vi "Gitlab OAuth Test.vi"() -> ()   [LabVIEW 2013]
uses:
  source/Oauth2/Oauth2.lvclass/Oauth2.ctl
  source/Oauth2/Read RefreshToken.vi
  source/Oauth2/Read ExpiresIn.vi
  source/Oauth2/Read Redirect URI.vi
  source/Oauth2/Read scopes.vi
  <vilib>/dlg_ctls.llb/Space Constant.vi
  source/OAuthToken/Retrieve Element.vi
  source/Oauth2.GitLab/Read Created At.vi
  source/Oauth2.GitLab/Read Created Timestamp.vi
  source/Oauth2/Oauth2.lvclass
  source/Oauth2.GitLab/Oauth2.GitLab.lvclass
  <vilib>/LabVIEW Open Source Project/OpenURI/uri/URI.lvclass
  <vilib>/httpClient/LabVIEWHTTPClient.lvlib
panel:
  out "REST API Error":errorcluster
  in  "Query API Version":bool
  in  "Refresh":bool
  in  "Authorize":bool
  out "Gitlab Version":string
  out "HTTP Response Headers":string
  out "Redirect URI":string
  out "granted scopes":string[](array[string])
  out "Created At":u32
  out "Expires In":u32
  out "Refresh Token":string
  in  "GitLab Client Secret":string
  in  "GitLab Client ID":string
  out "GitLab Access Token":string
  out "Oauth Error":errorcluster
  in  "GitLab Authorization Server URI":string="https://gitlab.com"
  # "Gitlab Application API Access Example"
  # "G Open Source Project for LabVIEW\nhttps://github.com/LabVIEW-Open-Source/Oauth2"
  # "1- Get a Client ID and Client Secret from the application's admin. \n\n          * To access your own server, log into your site, create an application and set the access scope.\n             you want. \n          * This Oauth2.0 API uses the following redirect URL: http://localhost:58888/Oauth2/Redirect\n          * Record the client ID and client secret and fill in the fields below."
  # "2- Set the Gitlab Authorization server address, without the relative \"oauth/authorize\" path.\n         * If using Gitlab's cloud, the URI is \"https://gitlab.com\"\n         * With your own domain, it could be \"https://gitlab.example.com\" or something similar."
  # "0: Never expired"
  # "3- Get an Access Token. You will be redirected your Gitlab's Authorization Server URI\n              * Use the \"Get Access Token\" button on the top right of this page.\n\n4- Once you have authenticated yourself, you will receive an access token.\n              * Use the \"Refresh Token\" button to request a fresh token\n                       OR\n              * Use the Access Token to query the Gitlab API (example is to retrieve the Gitlab Version)"
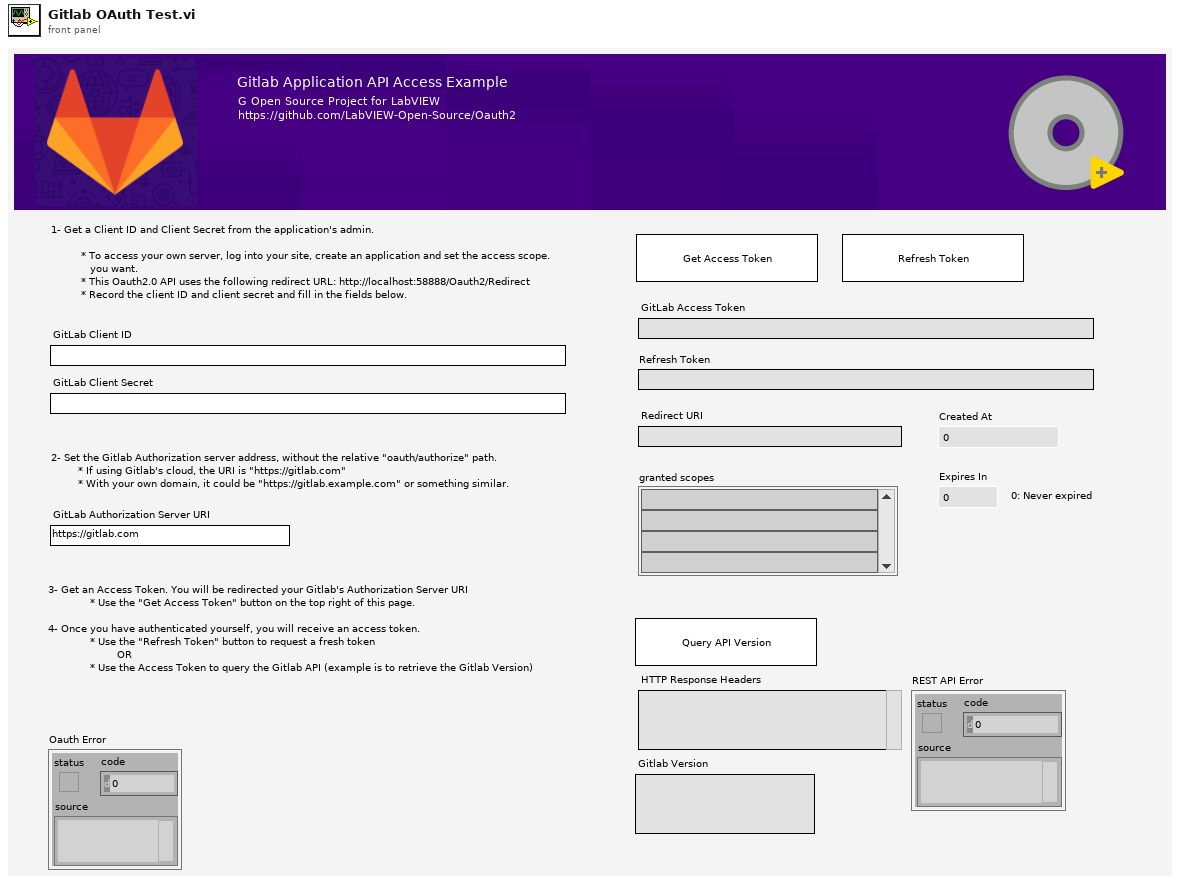
[diagram p1: front panel]
types:
  T1 = enum8{"Enabled", "Disabled", "Disabled and Grayed Out"}
  T2 = cluster{"Oauth2.GitLab":refnum<class "Oauth2.GitLab.lvclass">, "GitLab Authorization Server URI":string}
  T3 = typedef "LabVIEWHTTPClient.lvlib/ClientHandle.ctl" = refnum<k1>
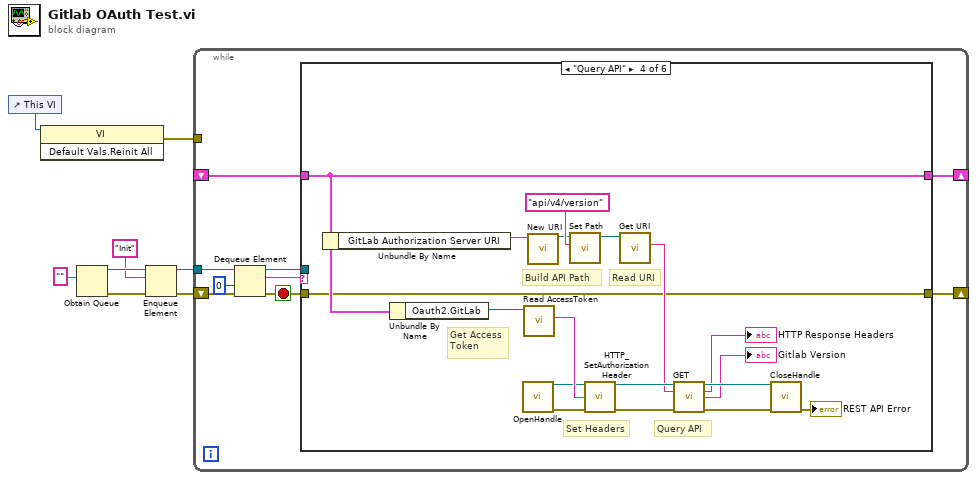
[diagram p0: block diagram]
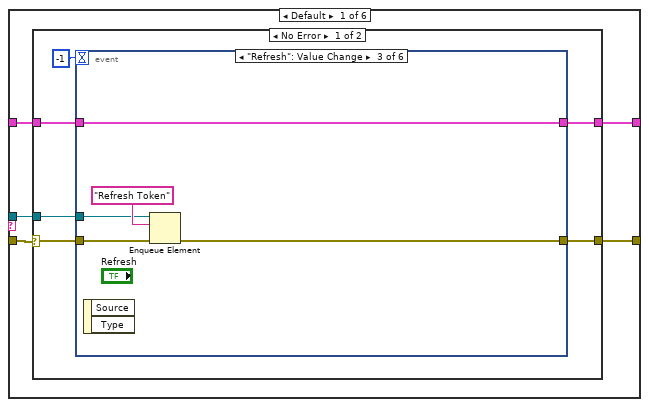
[diagram p2: hidden frame]
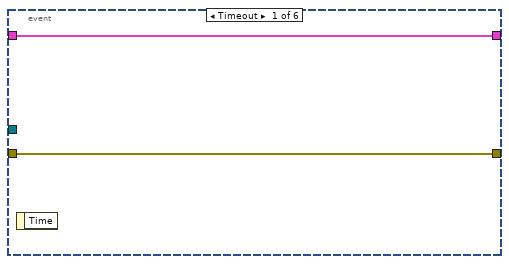
[diagram p3: hidden frame]
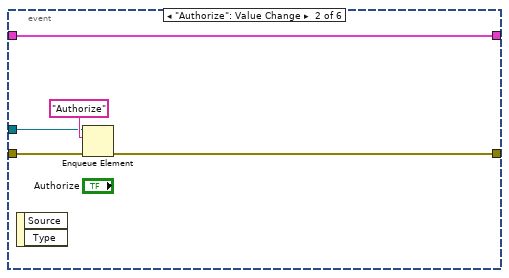
[diagram p4: hidden frame]
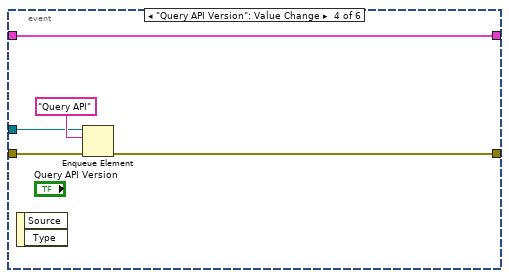
[diagram p5: hidden frame]
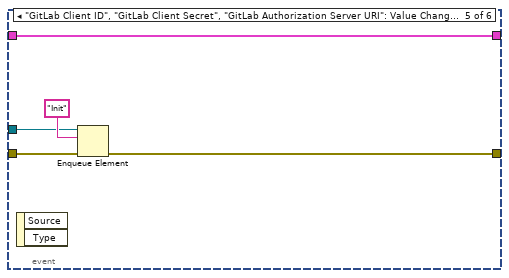
[diagram p6: hidden frame]
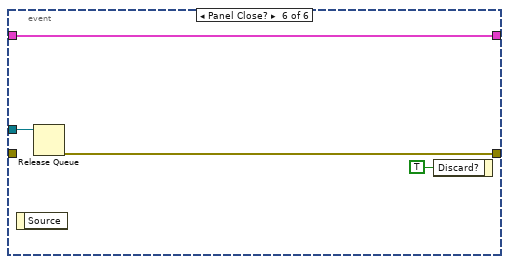
[diagram p7: hidden frame]
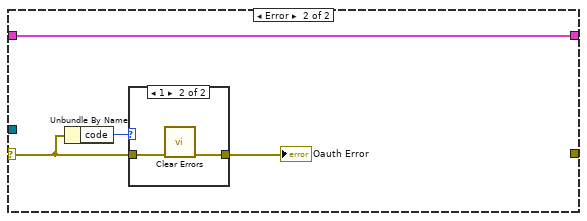
[diagram p8: hidden frame]
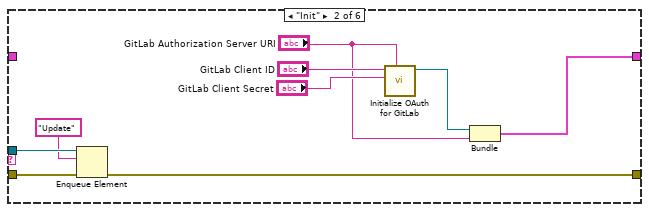
[diagram p10: hidden frame]
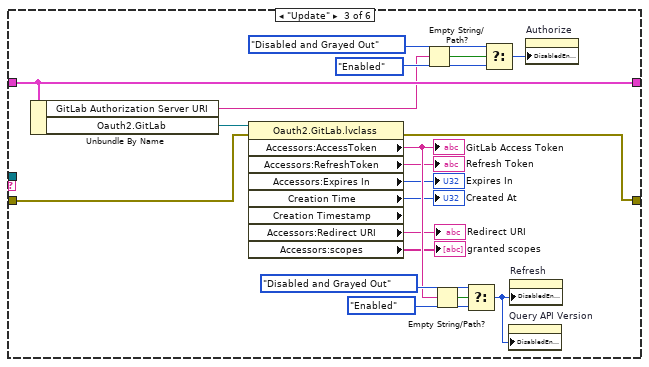
[diagram p11: hidden frame]
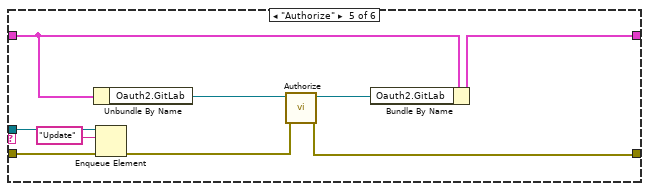
[diagram p12: hidden frame]
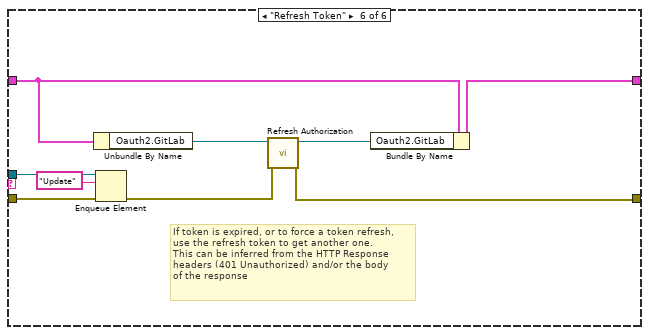
[diagram p13: hidden frame]
diagram:
  n1 = control-ref of="This VI"() -> (w2:refnum<vi>)
  n2 = invoke class="VI" method="Default Vals.Reinit All"(reference=w2) -> (error out=w1:errorcluster)  [unwired: 2 in, 2 out]
  n3 = Obtain Queue(element data type="") -> (queue out=w5:refnum<queue>, error out=w7:errorcluster)  [unwired: 4 in, 1 out]
  n4 = Enqueue Element(queue=w5, element="Init", error in (no error)=w7) -> (queue out=w4:refnum<queue>, error out=w6:errorcluster)  [unwired: 1 in, 1 out]
  n5 = while {
    tunnel: w4 -> [w17]
    shift-right: [w12] -> _
    shift-left: _ -> [w11]
    shift-right: [w9] -> _
    shift-left: w6 -> [w13]
    tunnel: w1 -> [_]
    stop <- w10 stop-if-true
    n6 = Dequeue Element(queue=w17, timeout in ms (-1)=0, error in (no error)=w13) -> (queue out=w14:refnum<queue>, element=w15:string, error out=w10:errorcluster)  [unwired: 1 out]
    n7 = case shown="\"Query API\"" w15 {
      tunnel: w14 -> [w22 w69 _ _ w110 w122]
      tunnel: [w21 w70 w89 w104 w112 w124] -> w12
      tunnel: w11 -> [w20 _ w89 w104 w113 w125]
      tunnel: w10 -> [w19 w66 w79 w92 w109 w121]
      tunnel: [w18 w67 w78 w92 w115 w117] -> w9
      frame Default {
        n8 = case shown="No Error" w19 {
          selector: w19 -> [w23 w57]
          tunnel: w22 -> [w27 _]
          tunnel: [w26 w58] -> w21
          tunnel: w20 -> [w25 w58]
          tunnel: [w24 _] -> w18
          frame No Error {
            n9 = event shown="[2] \"Refresh\": Value Change" {
              selector: _ -> [_ _ _ _ _ _]
              dyn-events: _ -> [_ _ _ _ _ _]
              timeout: -1 -> [_ _ _ _ _ _]
              tunnel: w27 -> [_ w34 w39 w44 w49 w54]
              tunnel: [w30 w32 w37 w42 w47 w52] -> w26
              tunnel: w25 -> [w30 w32 w37 w42 w47 w52]
              tunnel: [w29 w31 w36 w41 w46 w51] -> w24
              tunnel: w23 -> [w29 w33 w38 w43 w48 _]
              event Timeout {
                n10 = event-data() -> ()  [unwired: 1 in, 1 out]
              }
              event "Authorize": Value Change {
                n11 = event-data() -> ()  [unwired: 1 in, 2 out]
                n12 = Enqueue Element(queue=w34, element="Authorize", error in (no error)=w33) -> (error out=w31:errorcluster)  [unwired: 1 in, 2 out]
              }
              event "Refresh": Value Change {
                n13 = event-data() -> ()  [unwired: 1 in, 2 out]
                n14 = Enqueue Element(queue=w39, element="Refresh Token", error in (no error)=w38) -> (error out=w36:errorcluster)  [unwired: 1 in, 2 out]
              }
              event "Query API Version": Value Change {
                n15 = event-data() -> ()  [unwired: 1 in, 2 out]
                n16 = Enqueue Element(queue=w44, element="Query API", error in (no error)=w43) -> (error out=w41:errorcluster)  [unwired: 1 in, 2 out]
              }
              event "GitLab Client ID", "GitLab Client Secret", "GitLab Authorization Server URI": Value Change {
                n17 = event-data() -> ()  [unwired: 1 in, 2 out]
                n18 = Enqueue Element(queue=w49, element="Init", error in (no error)=w48) -> (error out=w46:errorcluster)  [unwired: 1 in, 2 out]
              }
              event Panel Close? {
                n19 = event-data() -> ()  [unwired: 1 in, 1 out]
                n20 = Release Queue(queue=w54) -> (error out=w51:errorcluster)  [unwired: 2 in, 2 out]
                n21 = event-data("Discard?"=TRUE) -> ()  [unwired: 1 in, 1 out]
              }
            }
          }
          frame Error {
            n22 = Unbundle By Name(w57) -> ("code"=w55:i32)
            n23 = case shown="1" w55 {
              tunnel: w57 -> [w59 w61]
              tunnel: [w59 w60] -> w56
              frame Default {
              }
              frame 1 {
                n24 = call <vilib>:"Clear Errors.vi"("error in (no error)"=w61) -> ("error out"=w60:errorcluster)  [unwired: 6 in]
              }
            }
            "Oauth Error" <- w56
          }
        }
      }
      frame "Init" {
        n25 = Enqueue Element(queue=w69, element="Update", error in (no error)=w66) -> (error out=w67:errorcluster)  [unwired: 1 in, 2 out]
        n26 = call "Initialize OAuth for GitLab.vi"("Authorization Server URI"="GitLab Authorization Server URI", "Client Secret"="GitLab Client Secret", "Client ID"="GitLab Client ID") -> ("Oauth2.GitLab"=w63:refnum<class "Oauth2.GitLab.lvclass">)  [unwired: 7 in, 1 out]
        n27 = Bundle("Oauth2.GitLab"=w63, "GitLab Authorization Server URI"="GitLab Authorization Server URI") -> (w70:T2)  [unwired: 1 in]
      }
      frame "Update" {
        n28 = Unbundle By Name(w89) -> ("GitLab Authorization Server URI"=w83:string, "Oauth2.GitLab"=w84:refnum<class "Oauth2.GitLab.lvclass">)
        n29 = property class="Oauth2.GitLab.lvclass" props=["Accessors:AccessToken", "Accessors:RefreshToken", "Accessors:Expires In", "Creation Time", "Creation Timestamp", "Accessors:Redirect URI", "Accessors:scopes"](reference=w84, error in=w79) -> (error out=w78:errorcluster, "Accessors:AccessToken"=w77:string, "Accessors:RefreshToken"=→"Refresh Token":string, "Accessors:Expires In"=→"Expires In":u32, "Creation Time"=→"Created At":u32, "Accessors:Redirect URI"=→"Redirect URI":string, "Accessors:scopes"=→"granted scopes":string[])  [unwired: 2 out]
        "GitLab Access Token" <- w77
        n30 = Empty String/Path?(string/path=w83) -> (empty?=w86:bool)
        n31 = Empty String/Path?(string/path=w77) -> (empty?=w82:bool)
        n32 = Select(t=T1."Disabled and Grayed Out" ("Disabled"), s=w82, f=T1."Enabled" ("Disabled")) -> (s? t:f=w71:T1)
        n33 = Select(t=T1."Disabled and Grayed Out" ("Disabled"), s=w86, f=T1."Enabled" ("Disabled")) -> (s? t:f=w85:T1)
        n34 = property on="Query API Version" class="Bool"("DisabledEnum"=w71) -> ()  [unwired: 2 in, 2 out]
        n35 = property on="Refresh" class="Bool"("DisabledEnum"=w71) -> ()  [unwired: 2 in, 2 out]
        n36 = property on="Authorize" class="Bool"("DisabledEnum"=w85) -> ()  [unwired: 2 in, 2 out]
      }
      frame "Query API" {
        # "Query API"
        # "Set Headers"
        # "Get Access\nToken"
        # "Read URI"
        # "Build API Path"
        n37 = Unbundle By Name(w104) -> ("GitLab Authorization Server URI"=w100:string)
        n38 = Unbundle By Name(w104) -> ("Oauth2.GitLab"=w105:refnum<class "Oauth2.GitLab.lvclass">)
        n39 = call <vilib>:"OpenHandle.vi"() -> ("client handle out"=w106:T3, "error out"=w97:errorcluster)  [unwired: 14 in]
        n40 = call "Read AccessToken.vi"("Oauth2 in"=w105) -> ("Access Token"=w107:string)  [unwired: 8 in, 2 out]
        n41 = call <vilib>:"New URI.vi"("URI"=w100) -> ("URI"=w101:refnum<class "URI.lvclass">)  [unwired: 9 in, 1 out]
        n42 = call <vilib>:"Set Path.vi"("path"="api/v4/version", "URI in"=w101) -> ("URI out"=w103:refnum<class "URI.lvclass">)  [unwired: 8 in, 1 out]
        n43 = call "HTTP_SetAuthorizationHeader.vi"("Client Handle"=w106, "Access Token"=w107, "error in (no error)"=w97) -> ("client handle dup"=w99:T3, "error out"=w96:errorcluster)  [unwired: 11 in]
        n44 = call <vilib>:"Get URI.vi"("URI in"=w103) -> ("URI String"=w98:string)  [unwired: 8 in, 2 out]
        n45 = call <vilib>:"GET.vi"("client handle"=w99, "url"=w98, "error in (no error)"=w96) -> ("client handle out"=w95:T3, "headers"=→"HTTP Response Headers":string, "body"=→"Gitlab Version":string, "error out"=w94:errorcluster)  [unwired: 9 in]
        n46 = call <vilib>:"CloseHandle.vi"("client handle"=w95, "error in (no error)"=w94) -> ("error out"=→"REST API Error":errorcluster)  [unwired: 13 in]
      }
      frame "Authorize" {
        n47 = Unbundle By Name(w113) -> ("Oauth2.GitLab"=w116:refnum<class "Oauth2.GitLab.lvclass">)
        n48 = Enqueue Element(queue=w110, element="Update", error in (no error)=w109) -> (error out=w108:errorcluster)  [unwired: 1 in, 2 out]
        n49 = call "Authorize.vi"("error in (no error)"=w108, "Oauth2 in"=w116) -> ("error out"=w115:errorcluster, "Oauth2 out"=w114:refnum<class "Oauth2.GitLab.lvclass">)  [unwired: 7 in, 1 out]
        n50 = Bundle By Name(cluster=w113, "Oauth2.GitLab"=w114) -> (w112:T2)
      }
      frame "Refresh Token" {
        # "If token is expired, or to force a token refresh, \nuse the refresh token to get another one.\nThis can be inferred from the HTTP Response\nheaders (401 Unauthorized) and/or the body\nof the response"
        n51 = Unbundle By Name(w125) -> ("Oauth2.GitLab"=w120:refnum<class "Oauth2.GitLab.lvclass">)
        n52 = Enqueue Element(queue=w122, element="Update", error in (no error)=w121) -> (error out=w118:errorcluster)  [unwired: 1 in, 2 out]
        n53 = call "Refresh Authorization.vi"("error in (no error)"=w118, "Oauth2 in"=w120) -> ("error out"=w117:errorcluster, "Oauth2 out"=w119:refnum<class "Oauth2.GitLab.lvclass">)  [unwired: 7 in, 1 out]
        n54 = Bundle By Name(cluster=w125, "Oauth2.GitLab"=w119) -> (w124:T2)
      }
    }
  }
